vi "Enter_Function.vi"(8 "error in (no error)":errorcluster, 10 "User Input":string, 11 "Data":T1) -> (0 "error out":errorcluster, 1 "Left Menu":T4, 2 "Right Menu":T4, 3 "Data Out":T1)   [LabVIEW 2019]
uses:
  controls/Data.ctl
  controls/Message Type.ctl
  controls/ATM Action.ctl
  controls/Read & Write File.ctl
  SubVIs/SubVI.lvlib
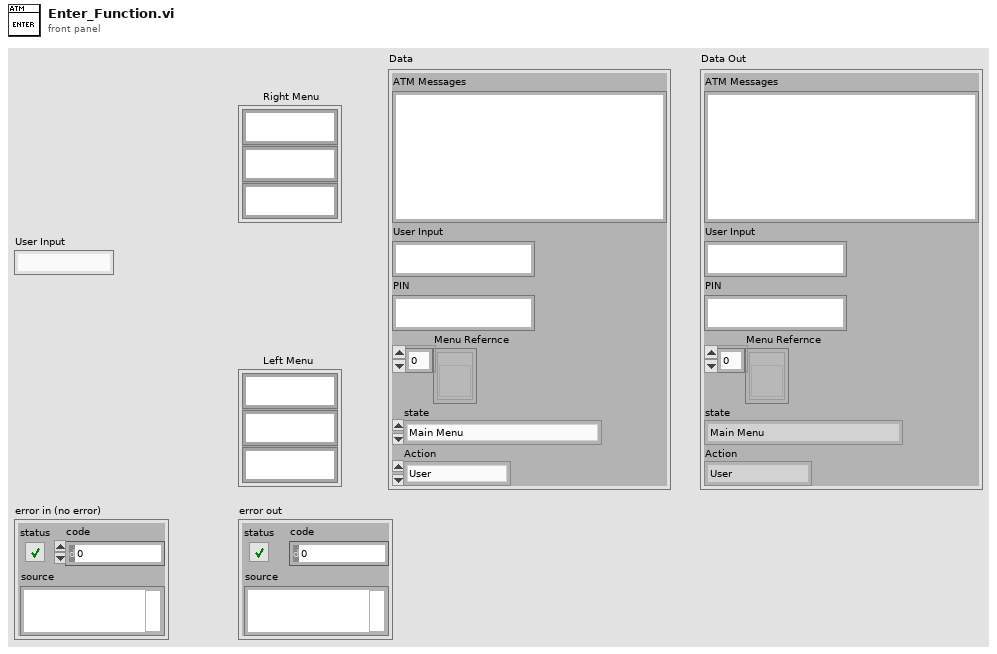
[diagram p1: front panel]
types:
  T1 = typedef "Data.ctl" = cluster{"ATM Messages":string, "User Input":string, "PIN":string, "Menu Refernce":refnum<vi>[], "state":T2, "Action":T3}
  T2 = typedef "Message Type.ctl" = enum16{"Main Menu", "Balance", "Withdrawal Complete", "Deposit Complete", "Welcome", "Account", "Session", "Deposit", "Withdraw", "Failed"}
  T3 = typedef "ATM Action.ctl" = enum16{"User", "Deposit", "Withdraw"}
  T4 = cluster{"RFS String":string, "RFS String 2":string, "RFS String 3":string}
  T5 = typedef "Read & Write File.ctl" = enum16{"Get Name", "Update Balance", "Init", "Get Balance"}
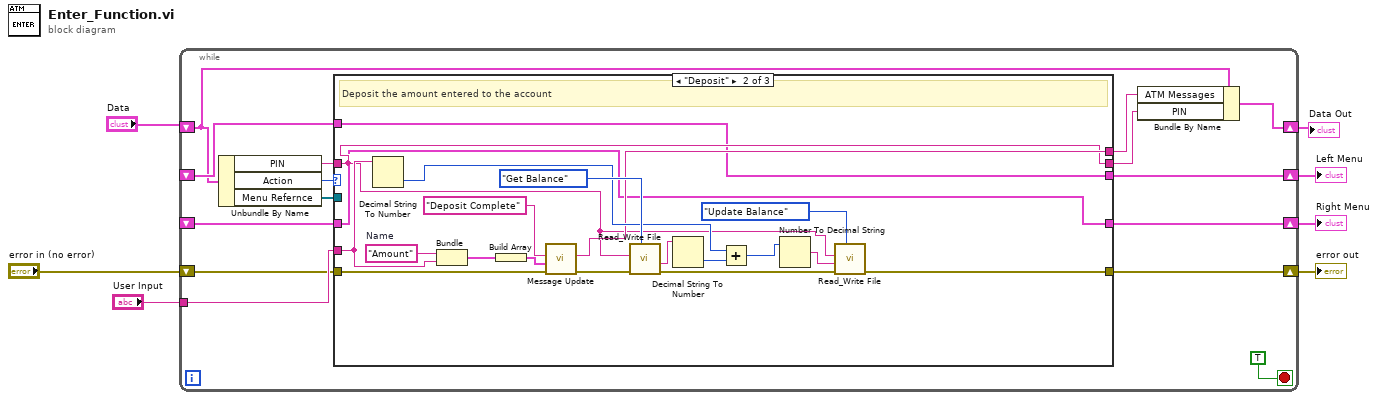
[diagram p0: block diagram]
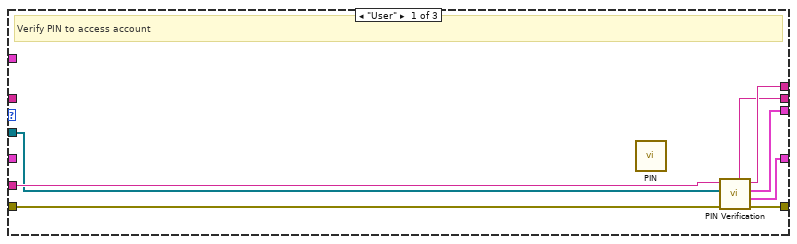
[diagram p2: hidden frame]
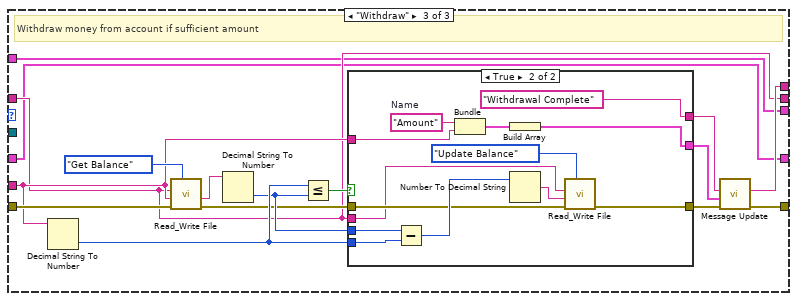
[diagram p3: hidden frame]
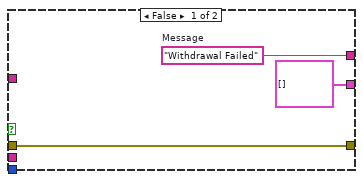
[diagram p4: hidden frame]
diagram:
  n1 = while {
    shift-right: [w20] -> w5
    shift-left: "error in (no error)" -> [w21]
    shift-right: [w18] -> w4
    shift-left: _ -> [w16]
    shift-right: [w19] -> w3
    shift-left: _ -> [w15]
    shift-right: [w9] -> w1
    shift-left: "Data" -> [w12]
    tunnel: "User Input" -> [w22]
    stop <- TRUE stop-if-true
    n2 = Unbundle By Name(w12) -> ("PIN"=w14:string, "Action"=w13:T3, "Menu Refernce"=w8:refnum<vi>[])
    n3 = case shown="\"Deposit\"" w13 {
      tunnel: [w30 w35 w55] -> w11
      tunnel: [w29 w36 w56] -> w20
      tunnel: [w28 w33 w53] -> w10
      tunnel: w21 -> [w27 w46 w63]
      tunnel: w22 -> [w26 w34 w54]
      tunnel: w14 -> [_ w33 w53]
      tunnel: [w24 w31 w51] -> w19
      tunnel: [w25 w32 w52] -> w18
      tunnel: w16 -> [_ w32 w52]
      tunnel: w15 -> [_ w31 w51]
      tunnel: w8 -> [w23 _ _]
      frame "User" {
        # "Verify PIN to access account"
        n4 = call "PIN.vi"() -> ()  [unwired: 7 in, 5 out]
        n5 = call "PIN Verification.vi"("error in (no error)"=w27, "Array"=w23, "PIN in"=w26) -> ("error out"=w29:errorcluster, "Right Menu"=w24:T4, "Left Menu"=w25:T4, "Message Out"=w30:string, "PIN"=w28:string)  [unwired: 4 in]
      }
      frame "Deposit" {
        w48 = "Amount"  # Name
        # "Deposit the amount entered to the account"
        n6 = Decimal String To Number(string=w34) -> (number=w41:i32)  [unwired: 2 in, 1 out]
        n7 = Bundle("Name"=w48, "User Input"=w34) -> (w49:cluster{"Name":string, "User Input":string})  [unwired: 1 in]
        n8 = Build Array(w49) -> (w47:cluster{"Name":string, "User Input":string}[])
        n9 = call "Message Update.vi"("error in (no error)"=w46, "Replace request"=w47, "Message type"="Deposit Complete" ("Message")) -> ("error out"=w44:errorcluster, "Message Out"=w35:string)  [unwired: 7 in]
        n10 = call "Read_Write File.vi"("Read/Write File"=Read_&_Write_File."Get Balance", "error in"=w44, "PIN_IN"=w33) -> ("error out"=w39:errorcluster, "Output Value"=w40:string)  [unwired: 5 in, 2 out]
        n11 = Decimal String To Number(string=w40) -> (number=w42:i32)  [unwired: 2 in, 1 out]
        n12 = Add(x=w41, y=w42) -> (x+y=w43:i32)
        n13 = Number To Decimal String(number=w43) -> (decimal integer string=w37:string)  [unwired: 1 in]
        n14 = call "Read_Write File.vi"("Read/Write File"=Read_&_Write_File."Update Balance", "error in"=w39, "User Input"=w37, "PIN_IN"=w33) -> ("error out"=w36:errorcluster)  [unwired: 4 in, 3 out]
      }
      frame "Withdraw" {
        # "Withdraw money from account if sufficient amount"
        n15 = Decimal String To Number(string=w54) -> (number=w60:i32)  [unwired: 2 in, 1 out]
        n16 = call "Read_Write File.vi"("Read/Write File"=Read_&_Write_File."Get Balance", "error in"=w63, "User Input"=w54, "PIN_IN"=w53) -> ("error out"=w58:errorcluster, "Output Value"=w62:string)  [unwired: 4 in, 2 out]
        n17 = Decimal String To Number(string=w62) -> (number=w59:i32)  [unwired: 2 in, 1 out]
        n18 = Less Or Equal?(x=w60, y=w59) -> (x <= y?=w61:bool)
        n19 = case shown="True" w61 {
          tunnel: [w68 "Withdrawal Complete" ("Message")] -> w66
          tunnel: [cluster{string, "User Input":string}[] [] w79] -> w65
          tunnel: w54 -> [_ w78]
          tunnel: w60 -> [_ w76]
          tunnel: w59 -> [_ w75]
          tunnel: w58 -> [w69 w72]
          tunnel: [w69 w71] -> w57
          tunnel: w53 -> [_ w70]
          frame False {
            w68 = "Withdrawal Failed"  # Message
          }
          frame True {
            w80 = "Amount"  # Name
            n20 = Subtract(x=w75, y=w76) -> (x-y=w77:i32)
            n21 = Bundle("Name"=w80, "User Input"=w78) -> (w81:cluster{"Name":string, "User Input":string})  [unwired: 1 in]
            n22 = Build Array(w81) -> (w79:cluster{"Name":string, "User Input":string}[])
            n23 = Number To Decimal String(number=w77) -> (decimal integer string=w73:string)  [unwired: 1 in]
            n24 = call "Read_Write File.vi"("Read/Write File"=Read_&_Write_File."Update Balance", "error in"=w72, "User Input"=w73, "PIN_IN"=w70) -> ("error out"=w71:errorcluster)  [unwired: 4 in, 3 out]
          }
        }
        n25 = call "Message Update.vi"("error in (no error)"=w57, "Replace request"=w65, "Message type"=w66) -> ("error out"=w56:errorcluster, "Message Out"=w55:string)  [unwired: 7 in]
      }
    }
    n26 = Bundle By Name(cluster=w12, "ATM Messages"=w11, "PIN"=w10) -> (w9:T1)
  }
  "error out" <- w5
  "Left Menu" <- w4
  "Right Menu" <- w3
  "Data Out" <- w1
